vi "1 port_Save Sweep Data to csv_ksENA.vi"(3 "Meas Type":string="QuickView_", 4 "PostTest Capacitance":dbl[](array[numeric]), 5 "Selected Exp Settings":T5={"Floor_Sweep_Stop_V"=36.0, "Resistance Threshold"=1.0, "Floor_Sweep_Start_V"=36.0, "Floor_Sweep_Step_V"=1.0, "Roof_Sweep_Stop_V"=36.0, "Roof_Sweep_Start_V"=36.0, "Roof_Sweep_Step_V"=1.0, "Meas Type"=enum."Floor", "Experiment Name"=""}, 6 "PreTest Capacitance":dbl[](array[numeric]), 7 "Filepath":path, 9 "ks5080A_Meaurements":T4, 10 "Date Cluster":T3, 11 "Test Information":T2={"Exp Name"="Cold Switching", "Lot"="0233A", "Wafer"="15", "Die Type"="L22", "Die X "="6", "Die Y"="8", "Exp"="1", "Die X_Y"="8"}) -> ()   [LabVIEW 2013]
uses:
  Controls/Date Control.ctl
  Controls/Test Information.ctl
  Controls/ks5080A_Measurements.ctl
  Controls/Individual User Inputs_Floor and Roof.ctl
  <vilib>/Utility/file.llb/Write To Spreadsheet File (string).vi
panel:
  in  "Tab Control":T1(tab)
  # "Test Settings"
  # "Calculation Settings"
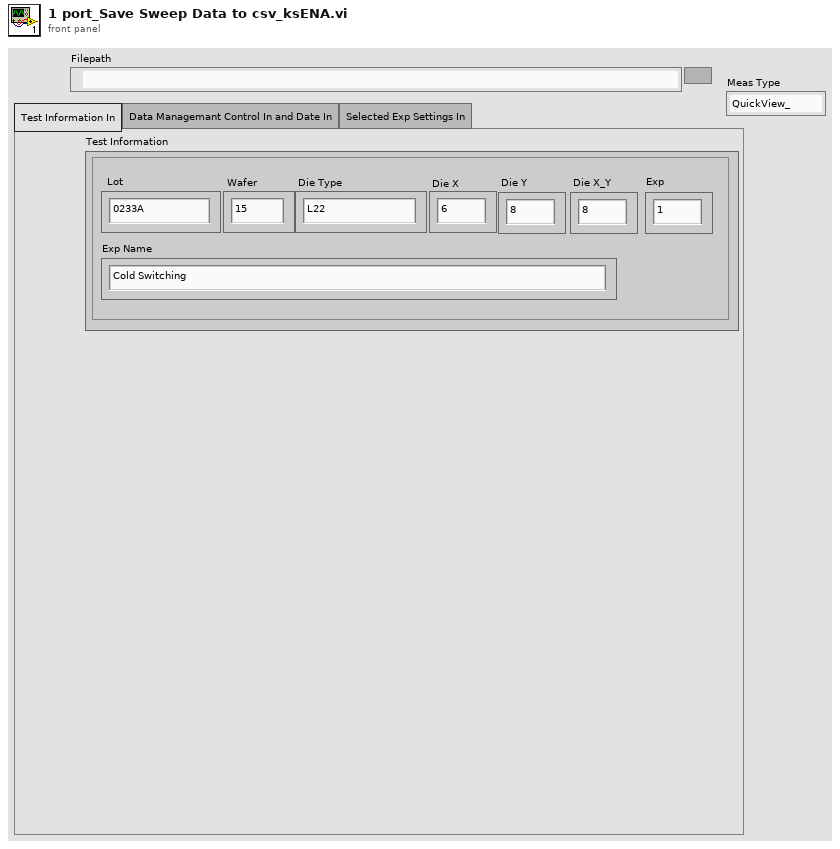
[diagram p1: front panel]
types:
  T1 = enum32{"Test Information In", "Data Managemant Control In and Date In", "Selected Exp Settings In"}
  T2 = typedef "Test Information.ctl" = cluster{"Exp Name":string, "Lot":string, "Wafer":string, "Die Type":string, "Die X ":string, "Die Y":string, "Exp":string, "Die X_Y":string}
  T3 = typedef "Date Control.ctl" = cluster{"Date":string, "Start Time":string, "Stop Time":string}
  T4 = typedef "ks5080A_Measurements.ctl" = cluster{"Bias_Sweep_Setting":dbl[], "Bias_voltage measurements":dbl[], "Bias_current measurements":dbl[], "P1_Capacitance":dbl[], "P2_Capacitance":dbl[], "DMM_Measurement_V":dbl[], "Contact_Source Current measurements":dbl[], "Contact_Sink Current measurements":dbl[], "Calculated_Resistance":dbl[], "P3_Capacitance":dbl[], "Port 1_S_parm":string[], "Port 2_S_parm":string[], "Port 3_S_parm":string[]}
  T5 = typedef "Individual User Inputs_Floor and Roof.ctl" = cluster{"Floor_Sweep_Stop_V":dbl, "Resistance Threshold":dbl, "Floor_Sweep_Start_V":dbl, "Floor_Sweep_Step_V":dbl, "Roof_Sweep_Stop_V":dbl, "Roof_Sweep_Start_V":dbl, "Roof_Sweep_Step_V":dbl, "Meas Type":enum16{"Floor", "Roof", "Floor and Roof"}, "Experiment Name":string}
  T6 = enum16{"open", "replace", "create", "open or create", "replace or create", "replace or create with confirmation"}
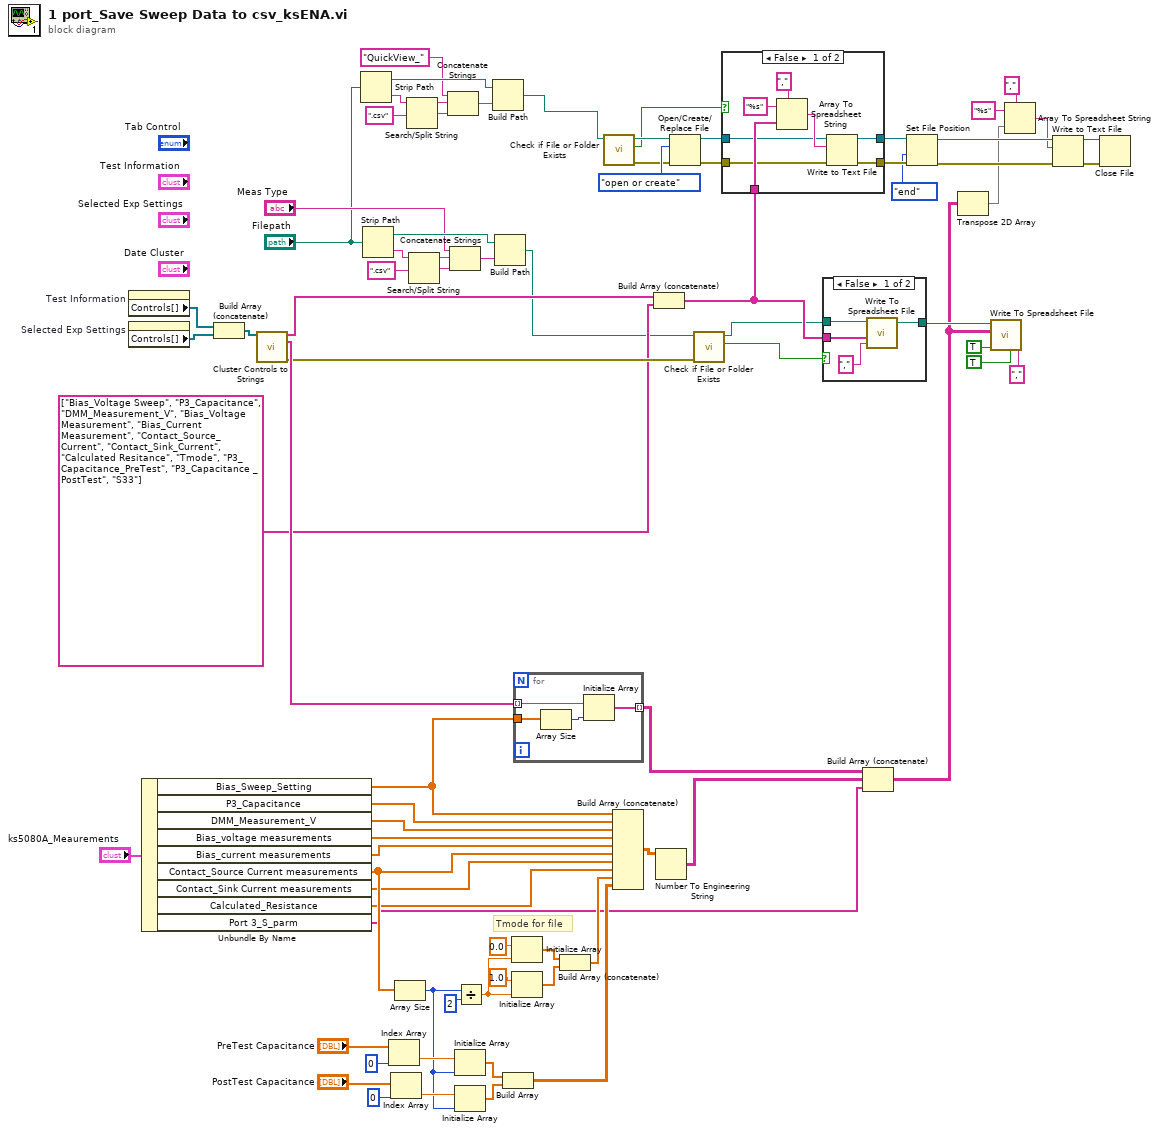
[diagram p0: block diagram]
diagram:
  # "Tmode for file"
  n1 = property on="Test Information" class="Clust (strict)"() -> ("Controls[]"=w79:refnum<vi>[])  [unwired: 2 in, 2 out]
  n2 = property on="Selected Exp Settings" class="Clust (strict)"() -> ("Controls[]"=w1:refnum<vi>[])  [unwired: 2 in, 2 out]
  n3 = Unbundle By Name("ks5080A_Meaurements") -> ("Bias_Sweep_Setting"=w56:dbl[], "P3_Capacitance"=w73:dbl[], "DMM_Measurement_V"=w72:dbl[], "Bias_voltage measurements"=w71:dbl[], "Bias_current measurements"=w70:dbl[], "Contact_Source Current measurements"=w69:dbl[], "Contact_Sink Current measurements"=w31:dbl[], "Calculated_Resistance"=w30:dbl[], "Port 3_S_parm"=w10:string[])
  n4 = Build Array (concatenate)(w79, w1) -> (w78:refnum<vi>[])
  n5 = call "Cluster Controls to Strings.vi"("Controls[]"=w78) -> ("Control Labels"=w58:string[], "Control Values"=w77:string[], "Error Out"=w57:errorcluster)  [unwired: 12 in]
  n6 = Strip Path(path="Filepath") -> (stripped path=w51:path, name=w54:string)
  n7 = Strip Path(path="Filepath") -> (stripped path=w14:path, name=w17:string)
  n8 = Index Array(array="PreTest Capacitance", index=0) -> (element=w26:dbl)
  n9 = Index Array(array="PostTest Capacitance", index=0) -> (element=w25:dbl)
  n10 = Array Size(array=w69) -> (size(s)=w24:i32)
  n11 = Search/Split String(string=w54, search string/char (-)=".csv" ("search string")) -> (substring before match=w49:string, match + rest of string=w52:string)  [unwired: 1 in, 1 out]
  n12 = Search/Split String(string=w17, search string/char (-)=".csv" ("search string")) -> (substring before match=w12:string, match + rest of string=w15:string)  [unwired: 1 in, 1 out]
  n13 = Concatenate Strings("QuickView_" ("search string"), w49, w52) -> (w50:string)
  n14 = Concatenate Strings("Meas Type", w12, w15) -> (w13:string)
  n15 = Initialize Array(w26, w24) -> (w23:dbl[])
  n16 = Initialize Array(w25, w24) -> (w22:dbl[])
  n17 = Divide(x=w24, y=2) -> (x/y=w75:dbl)
  n18 = Build Path(base path=w51, name or relative path=w50) -> (appended path=w7:path)
  n19 = Build Path(base path=w14, name or relative path=w13) -> (appended path=w3:path)
  n20 = Build Array(w23, w22) -> (w21:dbl[][])
  n21 = Initialize Array(0.0, w75) -> (w76:dbl[])
  n22 = Initialize Array(1.0, w75) -> (w66:dbl[])
  n23 = for {
    tunnel: w56 -> [w83]
    tunnel: w77 -> [w82] mode=indexing
    tunnel: [w80] -> w61 mode=indexing
    n24 = Array Size(array=w83) -> (size(s)=w81:i32)
    n25 = Initialize Array(w82, w81) -> (w80:string[])
  }
  n26 = Build Array (concatenate)(w76, w66) -> (w29:dbl[])
  n27 = call <vilib>:"Check if File or Folder Exists.vi"("path"=w7) -> ("error out"=w8:errorcluster, "file or folder exists?"=w5:bool, "dup path"=w6:path)  [unwired: 8 in]
  n28 = Build Array (concatenate)(w56, w73, w72, w71, w70, w69, w31, w30, w29, w21) -> (w59:dbl[][])
  n29 = Build Array (concatenate)(w58, string[] ["Bias_Voltage Sweep", "P3_Capacitance", "DMM_Measurement_V", "Bias_Voltage Measurement", "Bias_Current Measurement", "Contact_Source_Current", "Contact_Sink_Current", "Calculated Resitance", "Tmode", "P3_Capacitance_PreTest", "P3_Capacitance _PostTest", "S33"]) -> (w46:string[])
  n30 = Number To Engineering String(4:w59) -> (0:w60:string[][])  [unwired: 3 in]
  n31 = Open/Create/Replace File(file path (use dialog)=w6, error in=w8, operation (0:open)=T6."open or create") -> (refnum out=w45:refnum<file>, error out=w44:errorcluster)  [unwired: 3 in, 1 out]
  n32 = call <vilib>:"Check if File or Folder Exists.vi"("error in (no error)"=w57, "path"=w3) -> ("file or folder exists?"=w47:bool, "dup path"=w2:path)  [unwired: 7 in, 1 out]
  n33 = case shown="False" w5 {
    tunnel: w46 -> [w89 _]
    tunnel: w45 -> [w87 w93]
    tunnel: w44 -> [w86 w92]
    tunnel: [w85 w92] -> w42
    tunnel: [w84 w93] -> w43
    frame False {
      n34 = Array To Spreadsheet String(delimiter (Tab)="," ("delimiter (\\t)"), array=w89, 3:"%s" ("format string")) -> (spreadsheet string=w88:string)
      n35 = Write to Text File(file (use dialog)=w87, text=w88, error in=w86) -> (refnum out=w84:refnum<file>, error out=w85:errorcluster)  [unwired: 1 in, 1 out]
    }
    frame True {
    }
  }
  n36 = case shown="False" w47 {
    tunnel: w2 -> [w97 w98]
    tunnel: w46 -> [w96 _]
    tunnel: [w94 w98] -> w65
    frame False {
      n37 = call-poly <vilib>:"Write To Spreadsheet File.vi"("delimiter (\\t)"="," ("delimiter (\\t)"), "1D data"=w96, "file path (dialog if empty)"=w97) -> ("new file path (Not A Path if cancelled)"=w94:path)  [unwired: 5 in]
    }
    frame True {
    }
  }
  n38 = Build Array (concatenate)(w61, w60, w10) -> (w33:string[][])
  n39 = Set File Position(refnum=w43, from (0:start)=enum16{"start", "end", "current"}."end", error in=w42) -> (refnum out=w37:refnum<file>, error out=w38:errorcluster)  [unwired: 1 in]
  n40 = Transpose 2D Array(2D array=w33) -> (transposed array=w32:string[][])
  n41 = call-poly <vilib>:"Write To Spreadsheet File.vi"("delimiter (\\t)"="," ("delimiter (\\t)"), "transpose? (no:F)"=TRUE, "append to file? (new file:F)"=TRUE, "2D data"=w33, "file path (dialog if empty)"=w65) -> ()  [unwired: 3 in, 1 out]
  n42 = Array To Spreadsheet String(delimiter (Tab)="," ("delimiter (\\t)"), array=w32, 3:"%s" ("format string")) -> (spreadsheet string=w36:string)
  n43 = Write to Text File(file (use dialog)=w37, text=w36, error in=w38) -> (refnum out=w34:refnum<file>, error out=w35:errorcluster)  [unwired: 1 in, 1 out]
  n44 = Close File(refnum=w34, error in=w35) -> ()  [unwired: 2 out]
